vi "string_to_pstring_bytes.vi"(11 "string":string) -> (3 "PString Bytes":refnum<class "Bytes.lvclass">)   [LabVIEW 2020, in "variant.lvlib" / "variant.lvclass"]
uses:
  variant.lvclass
  Bytes/Bytes.lvclass
  Bytes/Bytes.lvclass/Bytes.ctl
  cb65cb49-3d91-4f6c-ab2a-423c4f682001.vi
  Bytes/from_byte_array.vi
  variant.lvclass/variant.ctl
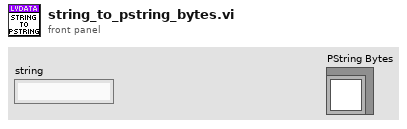
[diagram p1: front panel]
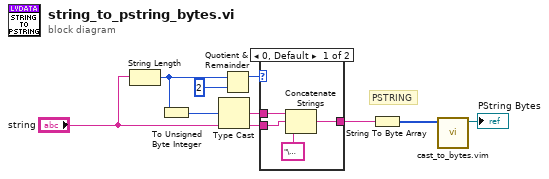
[diagram p0: block diagram]
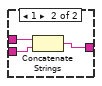
[diagram p2: hidden frame]
diagram:
  # "PSTRING"
  n1 = String Length(string="string") -> (length=w5:i32)
  n2 = To Unsigned Byte Integer(number=w5) -> (unsigned 8bit integer=w6:u8)
  n3 = Type Cast(x=w6) -> (*(type *) &x=w7:string)  [unwired: 1 in]
  n4 = Quotient & Remainder(x=w5, y=2) -> (x-y*floor(x/y)=w4:i32)  [unwired: 1 out]
  n5 = case shown="0, Default" w4 {
    tunnel: [w13 w14] -> w8
    tunnel: "string" -> [w12 w15]
    tunnel: w7 -> [w10 w16]
    frame 0, Default {
      n6 = Concatenate Strings(w10, w12, "\u0000" ("Substring")) -> (w13:string)
    }
    frame 1 {
      n7 = Concatenate Strings(w16, w15) -> (w14:string)
    }
  }
  n8 = String To Byte Array(string=w8) -> (unsigned byte array=w2:u8[])
  n9 = call "cast_to_bytes.vim"("anything"=w2) -> ("bytes"=→"PString Bytes":refnum<class "Bytes.lvclass">)  [unwired: 10 in]
